vi "Connect Const to Source.vi"(6 "Auto Route? (F)":bool, 7 "Auto Wire? (T)":bool, 8 "Error In":errorcluster, 9 "Source":refnum<vi>, 11 "Const in":refnum<vi>) -> (0 "Error Out":errorcluster, 3 "Const out":refnum<vi>)   [LabVIEW 2019, in "VI Scripting Utilities.lvlib"]
uses:
  VI Scripting Utilities.lvlib
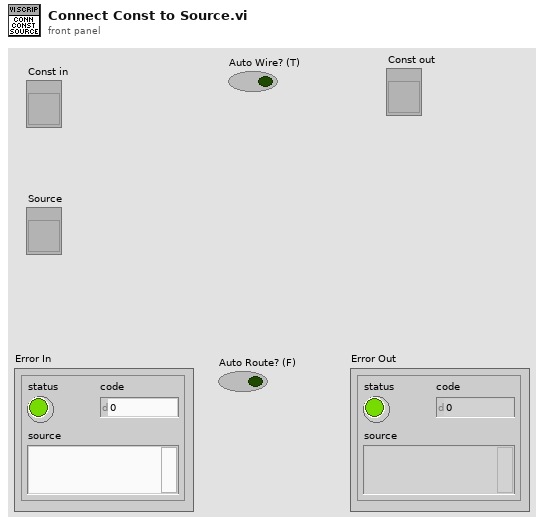
[diagram p1: front panel]
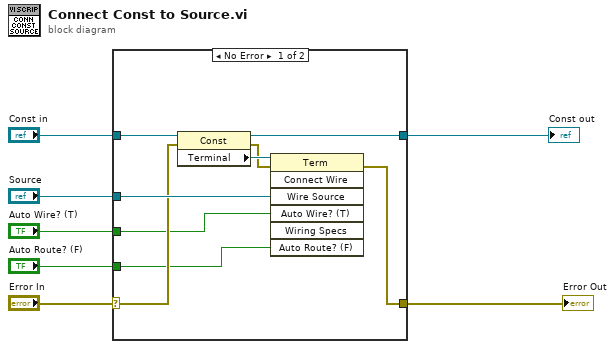
[diagram p0: block diagram]
diagram:
  n1 = case shown="No Error" "Error In" {
    selector: "Error In" -> [w13 w18]
    tunnel: "Const in" -> [w15 w17]
    tunnel: "Source" -> [w14 _]
    tunnel: [w11 w18] -> w4
    tunnel: [w10 w17] -> w3
    tunnel: "Auto Wire? (T)" -> [w9 _]
    tunnel: "Auto Route? (F)" -> [w8 _]
    frame No Error {
      n2 = property class="Const"(reference=w15, error in=w13) -> (reference out=w10:refnum<vi>, error out=w12:errorcluster, "Terminal"=w16:refnum<vi>)
      n3 = invoke class="Term" method="Connect Wire"(reference=w16, error in=w12, "Wire Source"=w14, "Auto Wire? (T)"=w9, "Auto Route? (F)"=w8) -> (error out=w11:errorcluster)  [unwired: 2 in, 6 out]
    }
    frame Error {
    }
  }
  "Error Out" <- w4
  "Const out" <- w3
